vi "Read Configuration.vi"(11 "error in (no error)":errorcluster) -> (3 "PythonPath":string, 4 "PythonVersion":string, 6 "server_api_key":string, 8 "server_url":string, 10 "workspace_name":string, 15 "error out":errorcluster)   [LabVIEW 2021, in "Measurement Builder.lvlib"]
uses:
  Measurement Builder.lvlib
  <vilib>/Utility/config.llb/Read Key (String).vi
  Path Functions/Path Functions.lvlib
  <vilib>/Utility/config.llb/NI_LVConfig.lvlib
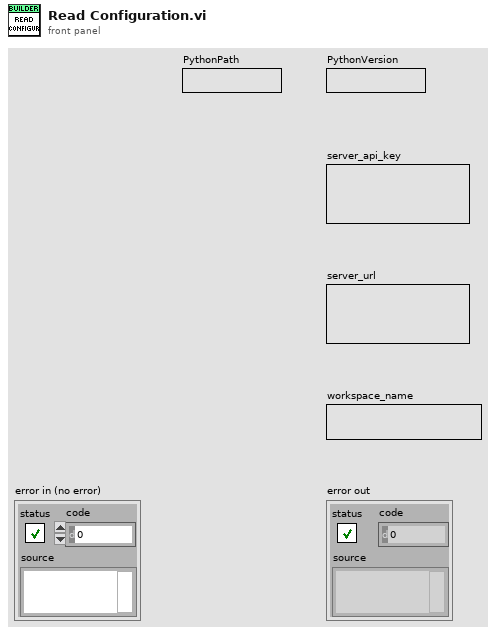
[diagram p1: front panel]
types:
  T1 = typedef "NI_LVConfig.lvlib/Config Data RefNum.ctl" = refnum<k1>
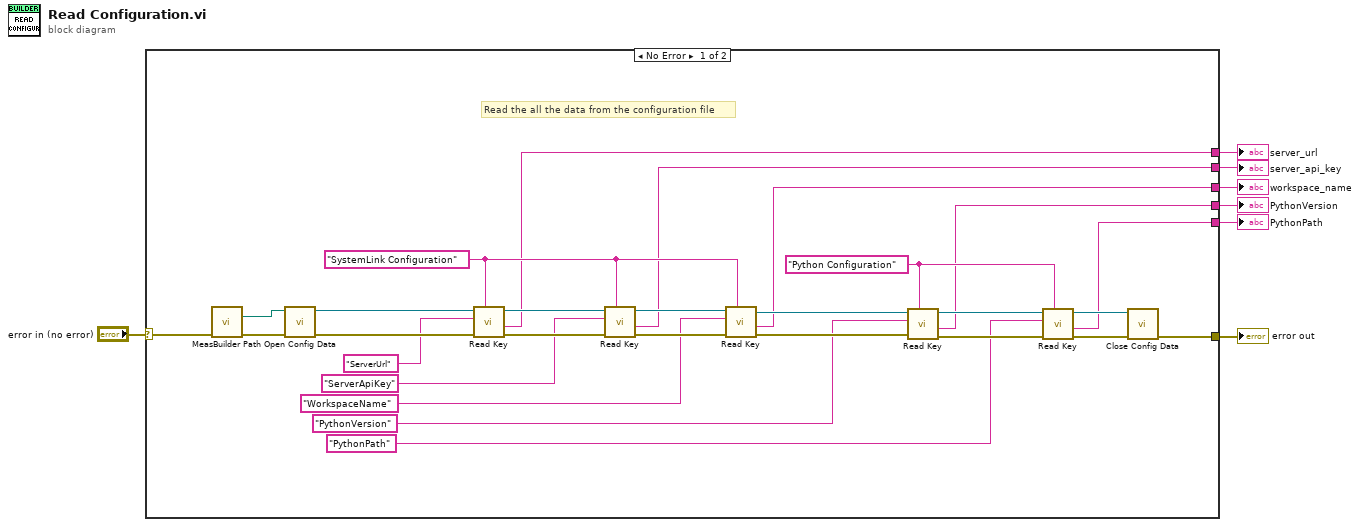
[diagram p0: block diagram]
diagram:
  n1 = case shown="No Error" "error in (no error)" {
    selector: "error in (no error)" -> [w35 w36]
    tunnel: [w15 w36] -> w7
    tunnel: [w14 _] -> w5
    tunnel: [w13 _] -> w4
    tunnel: [w12 _] -> w3
    tunnel: [w11 _] -> w2
    tunnel: [w10 _] -> w1
    frame No Error {
      w18 = "Python Configuration" ("section")
      w26 = "SystemLink Configuration" ("section")
      # "Read the all the data from the configuration file"
      n2 = call "MeasBuilder Path.vi"("error in (no error)"=w35) -> ("Config"=w34:path, "error out"=w33:errorcluster)  [unwired: 11 in, 2 out]
      n3 = call <vilib>:"Open Config Data.vi"("error in (no error)"=w33, "configuration file path"=w34) -> ("error out"=w32:errorcluster, "refnum"=w31:T1)  [unwired: 7 in, 1 out]
      n4 = call-poly <vilib>:"Read Key.vi"("section"=w26, "error in (no error)"=w32, "key"="ServerUrl", "refnum"=w31) -> ("error out"=w30:errorcluster, "value"=w14:string, "refnum out"=w28:T1)  [unwired: 4 in, 1 out]
      n5 = call-poly <vilib>:"Read Key.vi"("section"=w26, "error in (no error)"=w30, "key"="ServerApiKey", "refnum"=w28) -> ("error out"=w29:errorcluster, "value"=w13:string, "refnum out"=w27:T1)  [unwired: 4 in, 1 out]
      n6 = call-poly <vilib>:"Read Key.vi"("section"=w26, "error in (no error)"=w29, "key"="WorkspaceName", "refnum"=w27) -> ("error out"=w22:errorcluster, "value"=w12:string, "refnum out"=w21:T1)  [unwired: 4 in, 1 out]
      n7 = call-poly <vilib>:"Read Key.vi"("section"=w18, "error in (no error)"=w22, "key"="PythonVersion", "refnum"=w21) -> ("error out"=w20:errorcluster, "value"=w11:string, "refnum out"=w19:T1)  [unwired: 4 in, 1 out]
      n8 = call-poly <vilib>:"Read Key.vi"("section"=w18, "error in (no error)"=w20, "key"="PythonPath", "refnum"=w19) -> ("error out"=w17:errorcluster, "value"=w10:string, "refnum out"=w16:T1)  [unwired: 4 in, 1 out]
      n9 = call <vilib>:"Close Config Data.vi"("error in (no error)"=w17, "refnum"=w16) -> ("error out"=w15:errorcluster)  [unwired: 8 in, 1 out]
    }
    frame Error {
    }
  }
  "error out" <- w7
  "server_url" <- w5
  "server_api_key" <- w4
  "workspace_name" <- w3
  "PythonVersion" <- w2
  "PythonPath" <- w1
